vi "_PIM Tree.vi"   [LabVIEW 2011]
uses:
  LIB/PIM Version.vi
panel:
  # "Summitek PIM Test Tree\nSee Diagram"
types:
  T1 = typedef "OGAB Version.ctl" = cluster{"Version":string, "Build Number":u32, "Build Date/Time":dbl}
  T2 = typedef "Field Record.ctl" = cluster{"ixField":i32, "iSequenceOrder":i32, "sxFieldId":string, "sxSequenceId":string, "sDisplayName":string, "sValue":string, "sUnits":string, "nDataType":T3, "nNextItem":T4, "fSystem":bool, "fSystemValue":bool, "fRequired":bool, "fSetAtTest":bool, "fTestField":bool, "fDeleted":bool, "fIndexed":bool, "fFreeList":bool}
  T3 = typedef "Field DataTypes.ctl" = enum32{"text", "numeric", "list", "timestamp", "boolean"}
  T4 = typedef "Field NextItem.ctl" = enum32{"Reset", "Retain", "Auto-Increment"}
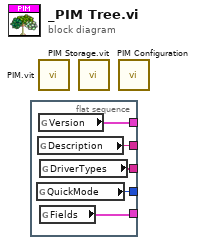
[diagram p0: block diagram]
diagram:
  n1 = flat-sequence {
    tunnel: [w5] -> _
    tunnel: [w4] -> _
    tunnel: [w3] -> _
    tunnel: [w2] -> _
    tunnel: [w1] -> _
    frame #0 {
      n2 = global read "PIM Version.vi" "QuickMode"() -> (w2:i32)
      n3 = global read "PIM Version.vi" "Description"() -> (w5:string)
      n4 = global read "PIM Version.vi" "Version"() -> (w4:T1)
      n5 = global read "PIM Version.vi" "DriverTypes"() -> (w3:string[])
      n6 = global read "PIM Version.vi" "Fields"() -> (w1:T2[])
    }
  }
  n7 = call "PIM.vit"() -> ()  [unwired: 4 in, 8 out]
  n8 = call "PIM Storage.vit"() -> ()  [unwired: 4 in, 8 out]
  n9 = call "PIM Configuration.vi"() -> ()  [unwired: 5 in, 7 out]
